vi "RUSHClimber.vi"(1 "In Cluster":T2) -> (0 "Out Cluster":T3)   [LabVIEW 2012]
panel:
  in  "DepDeadband":dbl=0.05
  in  "ClimbDepPGain":dbl=2.0
  in  "Rot Lowest POT pos":dbl=2.8
  in  "Rot Highest POT pot":dbl=3.17
  in  "Ext Highest POT pos":dbl=1.75
  in  "Ext Lowest POT pos":dbl=0.5
  out "ClimbConst":T1
  out "ClimbManualDep":dbl
  out "ClimbManualExt":dbl
  in  "Extension Speed":dbl=1.0
  in  "Deploy Speed":dbl=0.2
  in  "ExtDeadband":dbl=0.1
  # "For Local use only"
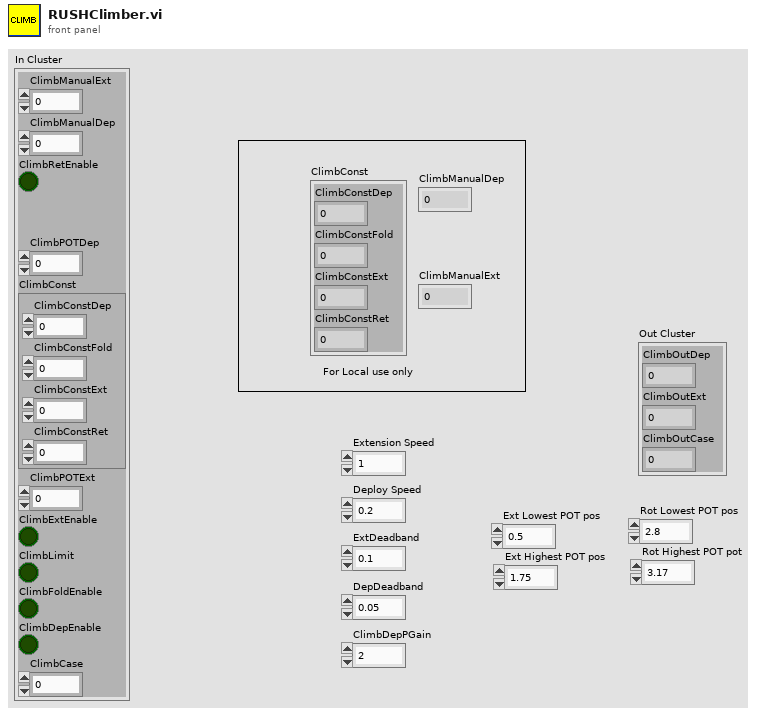
[diagram p1: front panel]
types:
  T1 = cluster{"ClimbConstDep":dbl, "ClimbConstFold":dbl, "ClimbConstExt":dbl, "ClimbConstRet":dbl}
  T2 = cluster{"ClimbManualExt":dbl, "ClimbManualDep":dbl, "ClimbRetEnable":bool, "ClimbPOTDep":dbl, "ClimbConst":cluster{"ClimbConstDep":dbl, "ClimbConstFold":dbl, "ClimbConstExt":dbl, "ClimbConstRet":dbl}, "ClimbPOTExt":dbl, "ClimbExtEnable":bool, "ClimbLimit":bool, "ClimbFoldEnable":bool, "ClimbDepEnable":bool, "ClimbCase":dbl}
  T3 = cluster{"ClimbOutDep":dbl, "ClimbOutExt":dbl, "ClimbOutCase":i32}
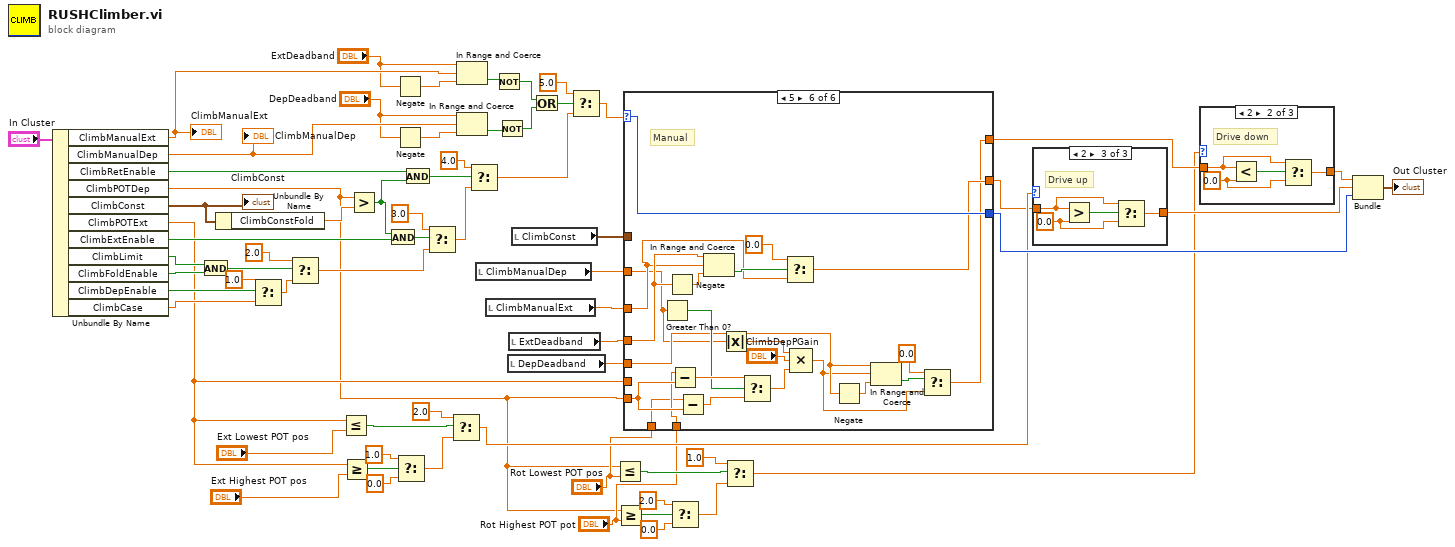
[diagram p0: block diagram]
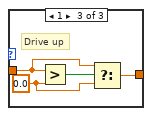
[diagram p3: hidden frame]
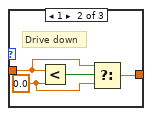
[diagram p5: hidden frame]
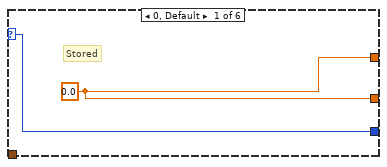
[diagram p6: hidden frame]
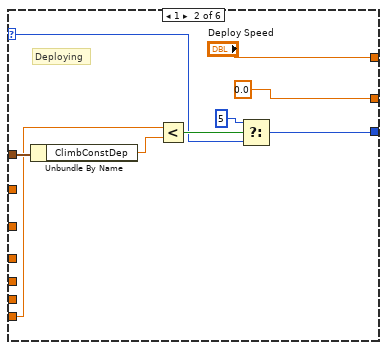
[diagram p7: hidden frame]
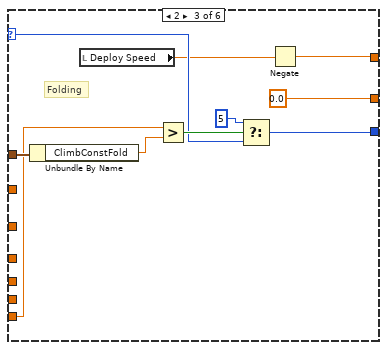
[diagram p8: hidden frame]
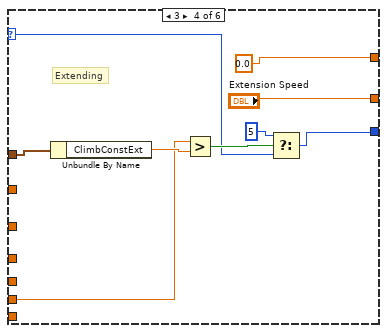
[diagram p9: hidden frame]
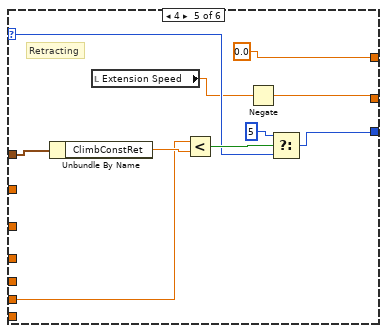
[diagram p10: hidden frame]
diagram:
  n1 = Unbundle By Name("In Cluster") -> ("ClimbManualExt"=w41:dbl, "ClimbManualDep"=w40:dbl, "ClimbRetEnable"=w39:bool, "ClimbPOTDep"=w4:dbl, "ClimbConst"=w38:T1, "ClimbPOTExt"=w20:dbl, "ClimbExtEnable"=w37:bool, "ClimbLimit"=w36:bool, "ClimbFoldEnable"=w35:bool, "ClimbDepEnable"=w32:bool, "ClimbCase"=w34:dbl)
  "ClimbManualExt" <- w41
  "ClimbManualDep" <- w40
  "ClimbConst" <- w38
  n2 = And(x=w36, y=w35) -> (x .and. y?=w63:bool)
  n3 = Unbundle By Name(w38) -> ("ClimbConstFold"=w53:dbl)
  n4 = Select(t=1.0, s=w32, f=w34) -> (s? t:f=w62:dbl)
  n5 = Select(t=2.0, s=w63, f=w62) -> (s? t:f=w55:dbl)
  n6 = Less Or Equal?(x=w20, y="Ext Lowest POT pos") -> (x <= y?=w22:bool)
  n7 = Greater Or Equal?(x=w20, y="Ext Highest POT pos") -> (x >= y?=w26:bool)
  n8 = Greater?(x=w4, y=w53) -> (0:w29:bool)
  n9 = And(x=w29, y=w37) -> (x .and. y?=w60:bool)
  n10 = Negate(x="ExtDeadband") -> (-x=w64:dbl)
  n11 = Negate(x="DepDeadband") -> (-x=w65:dbl)
  n12 = Select(t=1.0, s=w26, f=0.0) -> (s? t:f=w23:dbl)
  n13 = And(x=w39, y=w29) -> (x .and. y?=w56:bool)
  n14 = Select(t=3.0, s=w60, f=w55) -> (s? t:f=w58:dbl)
  n15 = Select(t=2.0, s=w22, f=w23) -> (s? t:f=w19:dbl)
  n16 = In Range and Coerce(upper limit="ExtDeadband", x=w41, lower limit=w64) -> (In Range?=w50:bool)  [unwired: 1 out]
  n17 = In Range and Coerce(upper limit="DepDeadband", x=w40, lower limit=w65) -> (In Range?=w51:bool)  [unwired: 1 out]
  n18 = Select(t=4.0, s=w56, f=w58) -> (s? t:f=w31:dbl)
  n19 = local read "ClimbManualDep"() -> (w7:dbl)
  n20 = local read "ClimbManualExt"() -> (w46:dbl)
  n21 = Not(x=w50) -> (.not. x?=w49:bool)
  n22 = Not(x=w51) -> (.not. x?=w48:bool)
  n23 = local read "DepDeadband"() -> (w1:dbl)
  n24 = local read "ExtDeadband"() -> (w45:dbl)
  n25 = local read "ClimbConst"() -> (w52:T1)
  n26 = Or(x=w49, y=w48) -> (x .or. y?=w47:bool)
  n27 = Select(t=5.0 ("f"), s=w47, f=w31) -> (s? t:f=w54:dbl)
  n28 = Less Or Equal?(x=w4, y="Rot Lowest POT pos") -> (x <= y?=w15:bool)
  n29 = Greater Or Equal?(x=w4, y="Rot Highest POT pot") -> (x >= y?=w11:bool)
  n30 = case shown="5" w54 {
    selector: w54 -> [w66 w73 w83 w92 w102 w124]
    tunnel: w52 -> [_ w76 w86 w91 w101 _]
    tunnel: [w66 w71 w81 w89 w99 w124] -> w44
    tunnel: [w67 "Deploy Speed" w78 0.0 ("Extend Speed") 0.0 ("Extend Speed") w115] -> w10
    tunnel: [w67 0.0 ("Extend Speed") 0.0 ("Extend Speed") "Extension Speed" w96 w116] -> w18
    tunnel: w7 -> [_ _ _ _ _ w107]
    tunnel: w46 -> [_ _ _ _ _ w117]
    tunnel: w45 -> [_ _ _ _ _ w127]
    tunnel: w20 -> [_ _ _ w90 w100 _]
    tunnel: "Rot Lowest POT pos" -> [_ _ _ _ _ w110]
    tunnel: "Rot Highest POT pot" -> [_ _ _ _ _ w111]
    tunnel: w4 -> [_ w68 w77 _ _ w112]
    tunnel: w1 -> [_ _ _ _ _ w119]
    frame 0, Default {
      w67 = 0.0
      # "Stored"
    }
    frame 1 {
      # "Deploying"
      n31 = Unbundle By Name(w76) -> ("ClimbConstDep"=w75:dbl)
      n32 = Less?(x=w68, y=w75) -> (x < y?=w74:bool)
      n33 = Select(t=5, s=w74, f=w73) -> (s? t:f=w71:i32)
    }
    frame 2 {
      # "Folding"
      n34 = Unbundle By Name(w86) -> ("ClimbConstFold"=w85:dbl)
      n35 = local read "Deploy Speed"() -> (w79:dbl)
      n36 = Greater?(x=w77, y=w85) -> (0:w84:bool)
      n37 = Select(t=5, s=w84, f=w83) -> (s? t:f=w81:i32)
      n38 = Negate(x=w79) -> (-x=w78:dbl)
    }
    frame 3 {
      # "Extending"
      n39 = Unbundle By Name(w91) -> ("ClimbConstExt"=w95:dbl)
      n40 = Greater?(x=w90, y=w95) -> (0:w94:bool)
      n41 = Select(t=5, s=w94, f=w92) -> (s? t:f=w89:i32)
    }
    frame 4 {
      # "Retracting"
      n42 = Unbundle By Name(w101) -> ("ClimbConstRet"=w105:dbl)
      n43 = local read "Extension Speed"() -> (w97:dbl)
      n44 = Less?(x=w100, y=w105) -> (x < y?=w104:bool)
      n45 = Negate(x=w97) -> (-x=w96:dbl)
      n46 = Select(t=5, s=w104, f=w102) -> (s? t:f=w99:i32)
    }
    frame 5 {
      # "Manual"
      n47 = Greater Than 0?(x=w107) -> (x > 0?=w122:bool)
      n48 = Negate(x=w127) -> (-x=w128:dbl)
      n49 = Subtract(x=w111, y=w112) -> (x-y=w123:dbl)
      n50 = Subtract(x=w110, y=w112) -> (x-y=w108:dbl)
      n51 = In Range and Coerce(upper limit=w127, x=w117, lower limit=w128) -> (In Range?=w126:bool)  [unwired: 1 out]
      n52 = Absolute Value(x=w107) -> (abs(x)=w113:dbl)
      n53 = Select(t=w123, s=w122, f=w108) -> (s? t:f=w109:dbl)
      n54 = Select(t=0.0, s=w126, f=w117) -> (s? t:f=w116:dbl)
      n55 = Compound Arithmetic op=MULTIPLY(w113, "ClimbDepPGain", w109) -> (w106:dbl)
      n56 = Negate(x=w119) -> (-x=w120:dbl)
      n57 = In Range and Coerce(upper limit=w119, x=w106, lower limit=w120) -> (In Range?=w121:bool)  [unwired: 1 out]
      n58 = Select(t=0.0, s=w121, f=w106) -> (s? t:f=w115:dbl)
    }
  }
  n59 = Select(t=2.0, s=w11, f=0.0) -> (s? t:f=w14:dbl)
  n60 = Select(t=1.0, s=w15, f=w14) -> (s? t:f=w8:dbl)
  n61 = case shown="2" w19 {
    tunnel: w18 -> [w129 w131 w135]
    tunnel: [w129 w130 w134] -> w17
    frame 0, Default {
      # "All good"
    }
    frame 1 {
      w132 = 0.0 ("y")
      # "Drive down"
      n62 = Less?(x=w131, y=w132) -> (x < y?=w133:bool)
      n63 = Select(t=w131, s=w133, f=w132) -> (s? t:f=w130:dbl)
    }
    frame 2 {
      w136 = 0.0 ("y")
      # "Drive up"
      n64 = Greater?(x=w135, y=w136) -> (0:w137:bool)
      n65 = Select(t=w135, s=w137, f=w136) -> (s? t:f=w134:dbl)
    }
  }
  n66 = case shown="2" w8 {
    tunnel: w10 -> [w138 w140 w144]
    tunnel: [w138 w139 w143] -> w9
    frame 0, Default {
      # "All good"
    }
    frame 2 {
      w141 = 0.0 ("y")
      # "Drive down"
      n67 = Less?(x=w140, y=w141) -> (x < y?=w142:bool)
      n68 = Select(t=w140, s=w142, f=w141) -> (s? t:f=w139:dbl)
    }
    frame 1 {
      w145 = 0.0 ("y")
      # "Drive up"
      n69 = Greater?(x=w144, y=w145) -> (0:w146:bool)
      n70 = Select(t=w144, s=w146, f=w145) -> (s? t:f=w143:dbl)
    }
  }
  n71 = Bundle("y"=w9, "y"=w17, "t"=w44) -> (→"Out Cluster":cluster{"y":dbl, "y":dbl, "t":i32})  [unwired: 1 in]
